vi "Imaq_find_ellipse.vi"(8 "error in (no error)":errorcluster, 9 "ROI1":T2, 10 "Image In":T4(plugin-control), 11 "ROI Descriptor":T3 {"Contours"."Type" items=["No Selection", "Point", "Line", "Rectangle", "Oval", "Polygon", "Freehand Region", "Annulus", "Unused2", "Unused3", "Broken Line", "Freehand Line", "Rotated Rectangle"]}) -> (0 "error out":errorcluster, 3 "New Reference":T1)   [LabVIEW 2019, in "Algorithm.lvclass"]
uses:
  FrameworkOverrides/Algorithm.lvclass
  <vilib>/vision/NI_Vision_Development_Module.lvlib
  <vilib>/vision/Pattern Matching.llb/IMAQ Match Range Setting.ctl
  <vilib>/vision/Shape Detection.llb/ShapeDetectionMatchOptions.ctl
  <vilib>/vision/Pattern Matching.llb/IMAQ Curve Parameters.ctl
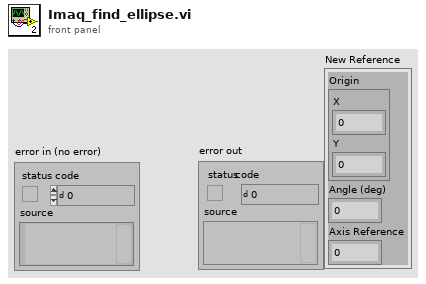
[diagram p1: front panel]
types:
  T1 = cluster{"Origin":cluster{"X":sgl, "Y":sgl}, "Angle (deg)":sgl, "Axis Reference":u32}
  T2 = cluster{"ROI":cluster{"Left":i32, "Top":i32, "Right":i32, "Bottom":i32, "Rotation":dbl}, "EdgeOptions":cluster{"EdgePolarity":i32, "KernelSize":i32, "Width":i32, "MinimumEdgeStrength":i32, "InterpolationType":i32, "DataProcessingMethod":i32}, "LineOptions":cluster{"NumberofLines":i32, "Type":i32, "MinScore":i32, "MaxScore":i32, "Orientation":i32, "AngleRange":i32, "AngleTolerance":i32, "StepSize":i32, "MinSNR":i32, "MinPoints":i32, "HoughIterations":i32}, "Process":i32, "StepSize":i32, "SearchDirection":i32, "CircleEdgeOptions":cluster{"SearchDirection":i32, "EdgeOptions":cluster{"EdgePolarity":i32, "KernelSize":i32, "Width":i32, "MinimumEdgeStrength":i32, "InterpolationType":i32, "DataProcessingMethod":i32}}, "CircleFitOptions":cluster{"Process":i32, "StepSize":i32, "MAxPixelRadius":i32}, "CircleSearchDirection":i32, "CurveParameters":cluster{"ExtractionMode":i32, "EdgeThreshold":i32, "EdgeFilterSize":i32, "MinLength":i32, "RowSearchStepSize":i32, "ColSearchStepSize":i32, "MaxEndpointGap":i32, "Closed":bool, "Subpixel":bool}, "MinimumMatchScore":i32, "CircleDescriptor":cluster{"MinRadius":i32, "MaxRadius":i32}, "EllipseDescriptor":cluster{"MinMajorRadius":i32, "MaxMajorRadius":i32, "MinMinorRadius":i32, "MaxMinorRadius":i32}, "ParallelLines":cluster{"First":i32, "Second":i32, "Third":i32}}
  T3 = cluster{"Global Rectangle":i32[], "Contours":cluster{"ID":enum32{"External", "Internal"}, "Type":u32, "Coordinates":i32[]}[]}
  T4 = typedef "IMAQ Image.ctl" = refnum<image>
  T5 = typedef "ShapeDetectionMatchOptions.ctl" = cluster{"Rotation":bool, "Scale":bool, "Occlusion":bool, "Range Settings":T6[]}
  T6 = typedef "IMAQ Match Range Setting.ctl" = cluster{"Match Constraints":u32, "Min":dbl, "Max":dbl}
  T7 = typedef "IMAQ Curve Parameters.ctl" = cluster{"Extraction Mode":u32, "Edge Threshold":i32, "Edge Filter Size":u32, "Min Length":i32, "Row Search Step Size":i32, "Col Search Step Size":i32, "Max Endpoint Gap":i32, "Closed":bool, "Subpixel":bool}
  T8 = cluster{"ExtractionMode":i32, "EdgeThreshold":i32, "EdgeFilterSize":i32, "MinLength":i32, "RowSearchStepSize":i32, "ColSearchStepSize":i32, "MaxEndpointGap":i32, "Closed":bool, "Subpixel":bool}
  T9 = cluster{"MinMajorRadius":i32, "MaxMajorRadius":i32, "MinMinorRadius":i32, "MaxMinorRadius":i32}
  T10 = cluster{"Position":cluster{"X":sgl, "Y":sgl}, "Angle":dbl, "Major Radius":dbl, "Minor Radius":dbl, "Score":dbl}[]
  T11 = cluster{"Position":cluster{"X":sgl, "Y":sgl}, "Angle":dbl, "Major Radius":dbl, "Minor Radius":dbl, "Score":dbl}
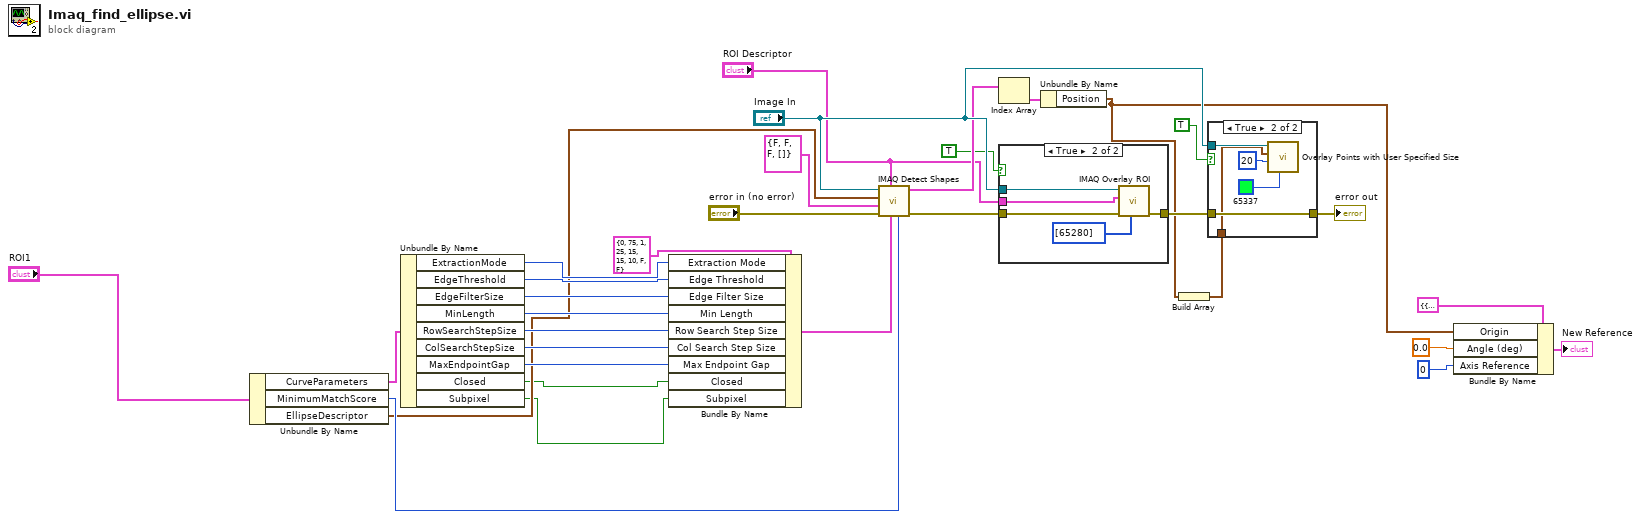
[diagram p0: block diagram]
diagram:
  n1 = Unbundle By Name("ROI1") -> ("CurveParameters"=w30:T8, "MinimumMatchScore"=w13:i32, "EllipseDescriptor"=w12:T9)
  n2 = Unbundle By Name(w30) -> ("ExtractionMode"=w23:i32, "EdgeThreshold"=w24:i32, "EdgeFilterSize"=w25:i32, "MinLength"=w26:i32, "RowSearchStepSize"=w27:i32, "ColSearchStepSize"=w28:i32, "MaxEndpointGap"=w29:i32, "Closed"=w9:bool, "Subpixel"=w8:bool)
  n3 = Bundle By Name(cluster=T7 {"Extraction Mode"=0, "Edge Threshold"=75, "Edge Filter Size"=1, "Min Length"=25, "Row Search Step Size"=15, "Col Search Step Size"=15, "Max Endpoint Gap"=10, "Closed"=FALSE, "Subpixel"=FALSE} ("Curve Parameters"), "Extraction Mode"=w23, "Edge Threshold"=w24, "Edge Filter Size"=w25, "Min Length"=w26, "Row Search Step Size"=w27, "Col Search Step Size"=w28, "Max Endpoint Gap"=w29, "Closed"=w9, "Subpixel"=w8) -> (w14:T7)
  n4 = call-poly "IMAQ Detect Shapes"("Minimum match score"=w13, "Curve Parameters"=w14, "ROI Descriptor"="ROI Descriptor", "error in (no error)"="error in (no error)", "Match Options"=T5 {"Rotation"=FALSE, "Scale"=FALSE, "Occlusion"=FALSE, "Range Settings"=[]}, "Ellipse Descriptor"=w12, "Image"="Image In") -> ("error out"=w18:errorcluster, "Ellipses"=w21:T10)  [unwired: 2 in, 1 out]
  n5 = Index Array(array=w21) -> (element=w20:T11)  [unwired: 1 in]
  n6 = case shown="True" TRUE {
    tunnel: w18 -> [w33 w37]
    tunnel: [w33 w36] -> w16
    tunnel: "Image In" -> [_ w38]
    tunnel: "ROI Descriptor" -> [_ w35]
    frame False {
    }
    frame True {
      n7 = call "IMAQ Overlay ROI"("Colors (Green)"=u32[] [65280], "error in (no error)"=w37, "ROI Descriptor"=w35, "Image"=w38) -> ("error out"=w36:errorcluster)  [unwired: 6 in, 1 out]
    }
  }
  n8 = Unbundle By Name(w20) -> ("Position"=w2:cluster{"X":sgl, "Y":sgl})
  n9 = Build Array(w2) -> (w6:cluster{"X":sgl, "Y":sgl}[])
  n10 = case shown="True" TRUE {
    tunnel: "Image In" -> [_ w43]
    tunnel: w16 -> [w39 w41]
    tunnel: [w39 w41] -> w15
    tunnel: w6 -> [_ w40]
    frame False {
    }
    frame True {
      n11 = call "Overlay Points with User Specified Size.vi"("Color"=u32 65337, "Point Diameter (5)"=u32 20, "Points"=w40, "Image In"=w43) -> ()  [unwired: 6 in, 2 out]
    }
  }
  "error out" <- w15
  n12 = Bundle By Name(cluster=T1 {"Origin"={"X"=0.0, "Y"=0.0}, "Angle (deg)"=0.0, "Axis Reference"=0} ("Coordinate System"), "Origin"=w2, "Angle (deg)"=sgl 0.0, "Axis Reference"=u32 0) -> (→"New Reference":T1)
